vi "NearestGlobal.vi"() -> ()   [LabVIEW 2016]
panel:
  out "nearest":dbl[](array[numeric])
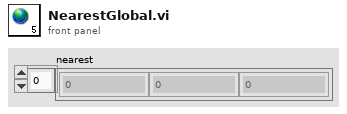
[diagram p1: front panel]
diagram:
